vi "FlatToRichni_bus_monitor_api_SetStreamingFilterReply.vi"(5 "OutputClusterType":T1, 11 "InputCluster":T3) -> (3 "OutputCluster":T1)   [LabVIEW 2025, in "bus_monitor_server.lvlib"]
uses:
  bus_monitor_server.lvlib
  ni_bus_monitor_api_SetStreamingFilterReply_Flat.ctl
  ni_bus_monitor_api_ErrorInfo_Flat.ctl
  ni_bus_monitor_api_SetStreamingFilterReply.ctl
  ni_bus_monitor_api_ErrorInfo.ctl
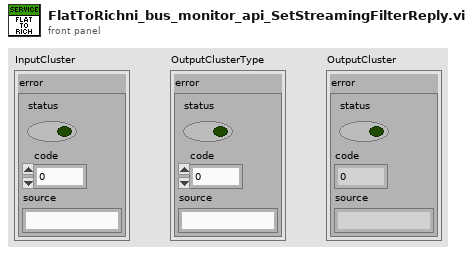
[diagram p1: front panel]
types:
  T1 = typedef "bus_monitor_server.lvlib/ni_bus_monitor_api_SetStreamingFilterReply.ctl" = cluster{"error":T2}
  T2 = typedef "bus_monitor_server.lvlib/ni_bus_monitor_api_ErrorInfo.ctl" = errorcluster
  T3 = typedef "bus_monitor_server.lvlib/ni_bus_monitor_api_SetStreamingFilterReply_Flat.ctl" = cluster{"error":T4}
  T4 = typedef "bus_monitor_server.lvlib/ni_bus_monitor_api_ErrorInfo_Flat.ctl" = errorcluster
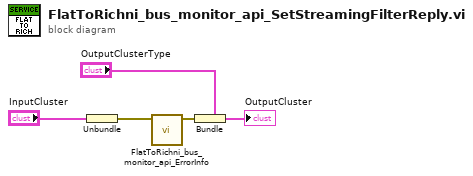
[diagram p0: block diagram]
diagram:
  n1 = Unbundle "Unbundle"("InputCluster") -> ("error"=w2:T4)
  n2 = call "FlatToRichni_bus_monitor_api_ErrorInfo.vi"("InputCluster"=w2) -> ("OutputCluster"=w1:T2)  [unwired: 10 in]
  n3 = Bundle "Bundle"(cluster="OutputClusterType", "error"=w1) -> (→"OutputCluster":T1)
